vi "setRemote.vi"(6 "error in (no error)":errorcluster, 8 "Remote Mode":bool=TRUE) -> (0 "error out":errorcluster)   [LabVIEW 2016]
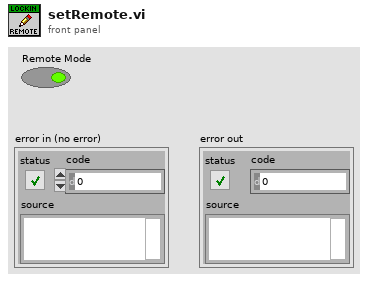
[diagram p1: front panel]
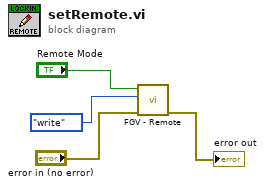
[diagram p0: block diagram]
diagram:
  n1 = call "FGV - Remote.vi"("error in"="error in (no error)", "Function"=enum16{"write", "read"}."write", "Remote Mode"="Remote Mode") -> ("error out"=→"error out":errorcluster)  [unwired: 3 in, 1 out]
